vi "Equalization.vi"(0 "data in":T1[](array[typedef])=[{"I"=0.0, "Q"=0.0, "overflow"=FALSE}, {"I"=0.0, "Q"=0.0, "overflow"=FALSE}], 9 "input valid":bool, 11 "gen in":refnum<class "niUSRP Tx DSP v2 FPGA.lvclass">) -> (4 "data out":T1[](array[typedef]), 10 "output valid":bool, 14 "ready for input":bool, 15 "gen out":refnum<class "niUSRP Tx DSP v2 FPGA.lvclass">)   [LabVIEW 2025, in "niUSRP Tx DSP v2 FPGA.lvclass"]
uses:
  niUSRP Tx DSP v2 FPGA.lvclass
  <instrlib>/_niInstr/DSP/v1/Shared/Public/IQ Data.ctl
  <instrlib>/_niInstr/DSP Control/Interface/v1/FPGA/Equalization/IQ 18-bit/Equalization Interface (IQ 18-bit).lvclass
  <instrlib>/_niInstr/Basic Elements/v1/FPGA/niInstr Basic Elements v1 FPGA.lvlib
  <instrlib>/_niInstr/DSP/v1/Shared/niInstr DSP v1 Shared.lvlib
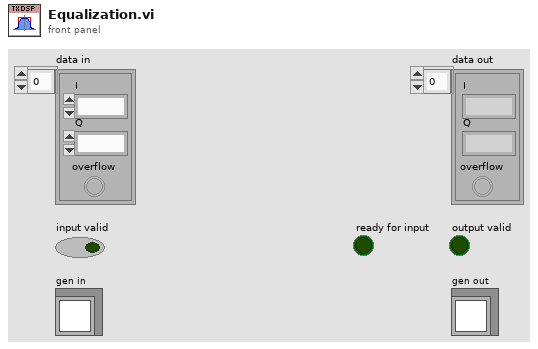
[diagram p1: front panel]
types:
  T1 = typedef "niInstr DSP v1 Shared.lvlib/IQ Data.ctl" = cluster{"I":fxp<+/-,18,1>, "Q":fxp<+/-,18,1>, "overflow":bool}
  T2 = typedef "niUSRP Tx DSP v2 FPGA.lvclass/Tx DSP Shared Registers.ctl" = cluster{"reset":refnum<k21>, "reset.done":refnum<k21>, "ignore overflows":refnum<k21>, "overflow":refnum<k21>, "overflow.clear":refnum<k21>, "pipeline delay":refnum<k21>, "group delay (output samples)":refnum<k21>, "blanking delay.data clock ticks":refnum<k21>, "dynamic delay.data clock ticks":refnum<k21>, "dynamic delay.samples":refnum<k21>, "bypass EQ":refnum<k21>, "inject idle into path":refnum<k21>, "TxDspEnabled":refnum<k21>}
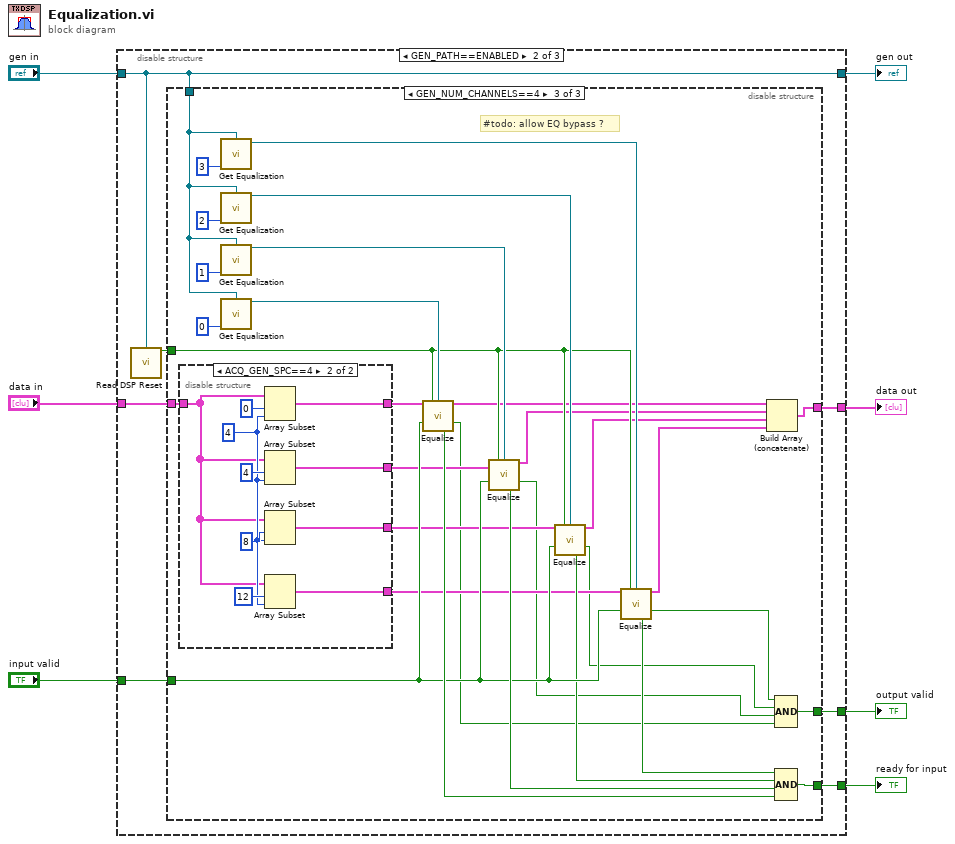
[diagram p0: block diagram]
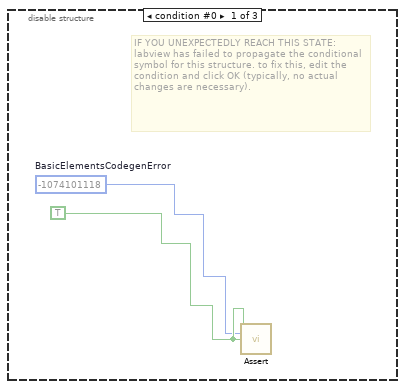
[diagram p2: hidden frame]
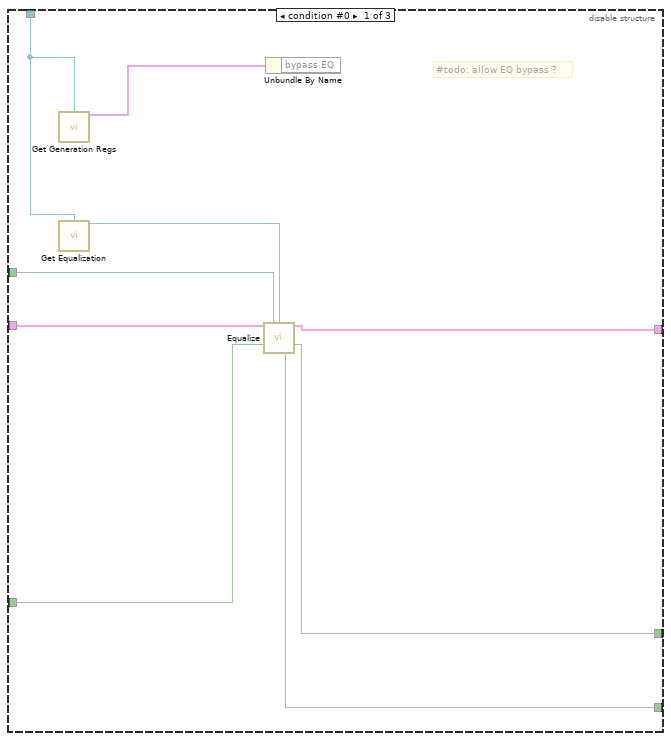
[diagram p3: hidden frame]
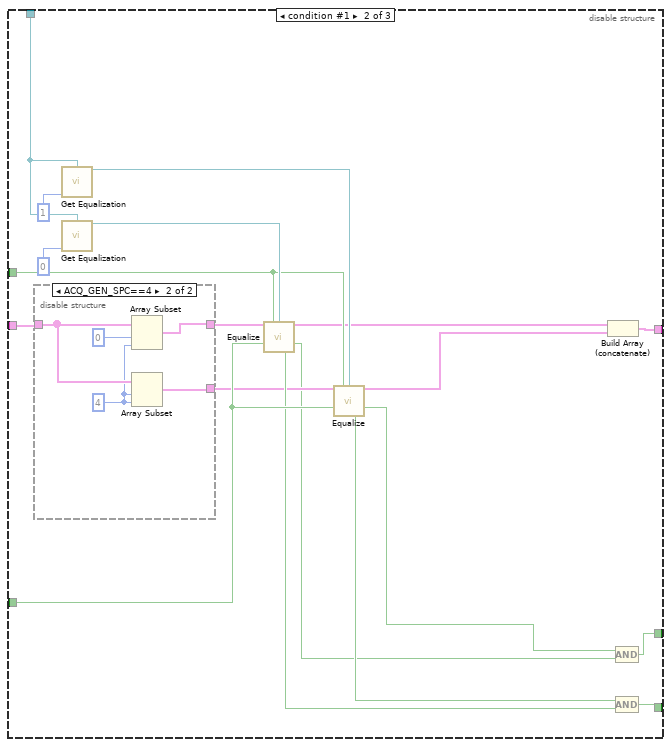
[diagram p4: hidden frame]
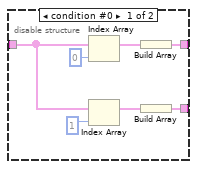
[diagram p5: hidden frame]
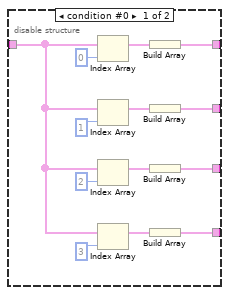
[diagram p6: hidden frame]
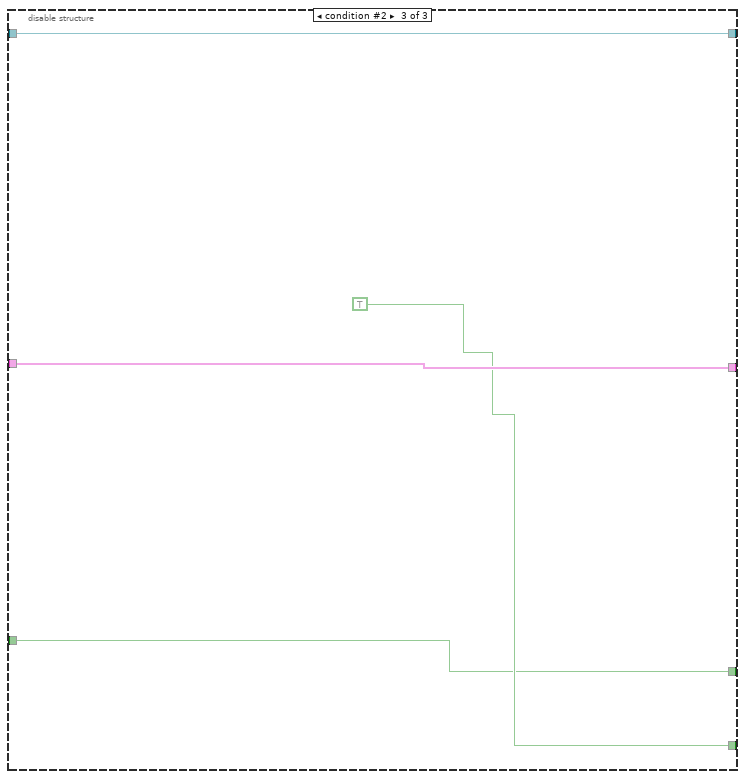
[diagram p7: hidden frame]
diagram:
  n1 = disable-structure shown="GEN_PATH==ENABLED" {
    disable-tunnel: [_ w10 w113] -> w7
    disable-tunnel: "input valid" -> [_ w15 w111]
    disable-tunnel: "gen in" -> [_ w11 w114]
    disable-tunnel: [_ w11 w114] -> w5
    disable-tunnel: [_ w14 w111] -> w4
    disable-tunnel: "data in" -> [_ w16 w113]
    disable-tunnel: [_ w12 TRUE ("ready for input")] -> w2
    frame condition #0 {
      w9 = TRUE ("assert")
      w8 = -1074101118  # BasicElementsCodegenError
      # "IF YOU UNEXPECTEDLY REACH THIS STATE:\nlabview has failed to propagate the conditional symbol for this structure. to fix this, edit the condition and click OK (typically, no actual changes are necessary)."
      n2 = call <instrlib>:"Assert.vi"("assert"=w9, "error code"=w8, "enable show error"=w9) -> ()  [unwired: 13 in]
    }
    frame condition #1 (active) {
      n3 = call-dynamic "Read DSP Reset.vi"("gen"=w11) -> ("dsp reset"=w13:bool)  [unwired: 14 in]
      n4 = disable-structure shown="GEN_NUM_CHANNELS==4" {
        disable-tunnel: w16 -> [w17 w32 w69]
        disable-tunnel: w15 -> [w25 w39 w75]
        disable-tunnel: [w24 w37 w82] -> w14
        disable-tunnel: w13 -> [w23 w33 w70]
        disable-tunnel: [w22 w34 w79] -> w12
        disable-tunnel: w11 -> [w19 w41 w76]
        disable-tunnel: [w18 w38 w83] -> w10
        frame condition #0 {
          # "#todo: allow EQ bypass ?"
          n5 = call-dynamic "Get Generation Regs.vi"("gen"=w19) -> ("dsp"=w20:T2)  [unwired: 14 in]
          n6 = call-dynamic "Get Equalization.vi"("gen"=w19) -> ("equalization"=w21:refnum<class "Equalization Interface (IQ 18-bit).lvclass">)  [unwired: 14 in]
          n7 = call-dynamic "Equalize.vi"("data in"=w17, "reset"=w23, "equalization"=w21, "input valid"=w25) -> ("data out"=w18:T1[], "output valid"=w24:bool, "ready for input"=w22:bool)  [unwired: 8 in, 1 out]
          n8 = Unbundle By Name(w20) -> ()  [unwired: 1 out]
        }
        frame condition #1 {
          n9 = disable-structure shown="ACQ_GEN_SPC==4" {
            disable-tunnel: w32 -> [w47 w54]
            disable-tunnel: [w46 w55] -> w31
            disable-tunnel: [w45 w53] -> w30
            frame condition #0 {
              n10 = Index Array(array=w47, index=0) -> (element=w51:T1)
              n11 = Index Array(array=w47, index=1) -> (element=w49:T1)
              n12 = Build Array(w51) -> (w46:T1[])
              n13 = Build Array(w49) -> (w45:T1[])
            }
            frame condition #1 (active) {
              w52 = 4 ("length")
              n14 = Array Subset(array=w54, index=0, length=w52) -> (w55:T1[])
              n15 = Array Subset(array=w54, index=w52, length=w52) -> (w53:T1[])
            }
          }
          n16 = call-dynamic "Get Equalization.vi"("gen"=w41, "ch"=u8 1) -> ("equalization"=w40:refnum<class "Equalization Interface (IQ 18-bit).lvclass">)  [unwired: 13 in]
          n17 = call-dynamic "Get Equalization.vi"("gen"=w41, "ch"=u8 0) -> ("equalization"=w44:refnum<class "Equalization Interface (IQ 18-bit).lvclass">)  [unwired: 13 in]
          n18 = call-dynamic "Equalize.vi"("data in"=w31, "reset"=w33, "equalization"=w44, "input valid"=w39) -> ("data out"=w29:T1[], "output valid"=w26:bool, "ready for input"=w36:bool)  [unwired: 8 in, 1 out]
          n19 = call-dynamic "Equalize.vi"("data in"=w30, "reset"=w33, "equalization"=w40, "input valid"=w39) -> ("data out"=w28:T1[], "output valid"=w27:bool, "ready for input"=w35:bool)  [unwired: 8 in, 1 out]
          n20 = Build Array (concatenate)(w29, w28) -> (w38:T1[])
          n21 = Compound Arithmetic op=AND(w27, w26) -> (w37:bool)
          n22 = Compound Arithmetic op=AND(w35, w36) -> (w34:bool)
        }
        frame condition #2 (active) {
          # "#todo: allow EQ bypass ?"
          n23 = disable-structure shown="ACQ_GEN_SPC==4" {
            disable-tunnel: [w96 w104] -> w68
            disable-tunnel: [w95 w103] -> w67
            disable-tunnel: [w94 w102] -> w66
            disable-tunnel: w69 -> [w89 w105]
            disable-tunnel: [w88 w101] -> w65
            frame condition #0 {
              n24 = Index Array(array=w89, index=0) -> (element=w100:T1)
              n25 = Index Array(array=w89, index=1) -> (element=w98:T1)
              n26 = Index Array(array=w89, index=2) -> (element=w90:T1)
              n27 = Index Array(array=w89, index=3) -> (element=w92:T1)
              n28 = Build Array(w100) -> (w96:T1[])
              n29 = Build Array(w98) -> (w95:T1[])
              n30 = Build Array(w90) -> (w94:T1[])
              n31 = Build Array(w92) -> (w88:T1[])
            }
            frame condition #1 (active) {
              w106 = 4 ("length")
              n32 = Array Subset(array=w105, index=0, length=w106) -> (w104:T1[])
              n33 = Array Subset(array=w105, index=4, length=w106) -> (w103:T1[])
              n34 = Array Subset(array=w105, index=8, length=w106) -> (w102:T1[])
              n35 = Array Subset(array=w105, index=12, length=w106) -> (w101:T1[])
            }
          }
          n36 = call-dynamic "Get Equalization.vi"("gen"=w76, "ch"=u8 3) -> ("equalization"=w73:refnum<class "Equalization Interface (IQ 18-bit).lvclass">)  [unwired: 13 in]
          n37 = call-dynamic "Get Equalization.vi"("gen"=w76, "ch"=u8 2) -> ("equalization"=w74:refnum<class "Equalization Interface (IQ 18-bit).lvclass">)  [unwired: 13 in]
          n38 = call-dynamic "Get Equalization.vi"("gen"=w76, "ch"=u8 1) -> ("equalization"=w84:refnum<class "Equalization Interface (IQ 18-bit).lvclass">)  [unwired: 13 in]
          n39 = call-dynamic "Get Equalization.vi"("gen"=w76, "ch"=u8 0) -> ("equalization"=w87:refnum<class "Equalization Interface (IQ 18-bit).lvclass">)  [unwired: 13 in]
          n40 = call-dynamic "Equalize.vi"("data in"=w68, "reset"=w70, "equalization"=w87, "input valid"=w75) -> ("data out"=w64:T1[], "output valid"=w57:bool, "ready for input"=w81:bool)  [unwired: 8 in, 1 out]
          n41 = call-dynamic "Equalize.vi"("data in"=w67, "reset"=w70, "equalization"=w84, "input valid"=w75) -> ("data out"=w63:T1[], "output valid"=w58:bool, "ready for input"=w80:bool)  [unwired: 8 in, 1 out]
          n42 = call-dynamic "Equalize.vi"("data in"=w66, "reset"=w70, "equalization"=w74, "input valid"=w75) -> ("data out"=w62:T1[], "output valid"=w59:bool, "ready for input"=w72:bool)  [unwired: 8 in, 1 out]
          n43 = call-dynamic "Equalize.vi"("data in"=w65, "reset"=w70, "equalization"=w73, "input valid"=w75) -> ("data out"=w61:T1[], "output valid"=w60:bool, "ready for input"=w71:bool)  [unwired: 8 in, 1 out]
          n44 = Build Array (concatenate)(w64, w63, w62, w61) -> (w83:T1[])
          n45 = Compound Arithmetic op=AND(w60, w59, w58, w57) -> (w82:bool)
          n46 = Compound Arithmetic op=AND(w71, w72, w80, w81) -> (w79:bool)
        }
      }
    }
    frame condition #2 {
    }
  }
  "data out" <- w7
  "output valid" <- w4
  "ready for input" <- w2
  "gen out" <- w5
